vi "REACTOR_COMUNICACIONES.vi"(8 "error in (no error)":errorcluster) -> (0 "error out":errorcluster, 1 "COMMS":T1={"Alicats"="COM4", "Alic"=TRUE, "eValve"="COM6", "eval"=TRUE, "Eurotherm"="COM8", "euro"=TRUE, "Cell GAS"="COM10", "cgas"=TRUE, "Cell H2S"="COM5", "ch2s"=TRUE}, 2 "Cancelled?":bool)   [LabVIEW 2017]
doc: "Use this template to create a dialog box. This template polls the state of the buttons on the front panel and does not use events. Use the Dialog Using Events template (not available in Base package) to create a dialog box with event handling."
uses:
  REACTOR_COMUNICACIONES.ctl
panel:
  in  "Alic":bool=TRUE
  in  "Euro":bool=TRUE
  in  "V4v":bool=TRUE
  in  "Alicats":refnum<visa-resource-name>="COM4"
  in  "Eurotherm":refnum<visa-resource-name>="COM6"
  in  "EV4Posic":refnum<visa-resource-name>="COM7"
  out "Enable":bool=TRUE
  out "Disable":bool
  in  "Cancel":bool
  in  "OK":bool
  # "Comunicaciones"
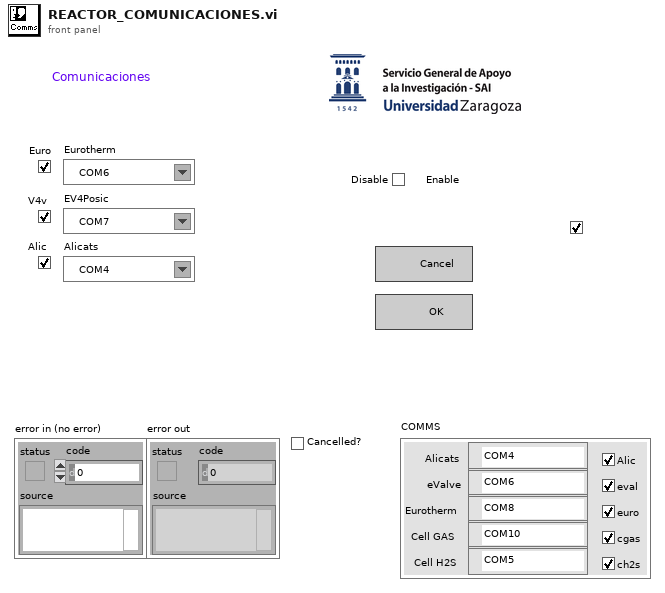
[diagram p1: front panel]
types:
  T1 = typedef "REACTOR_COMUNICACIONES.ctl" = cluster{"Alicats":refnum<visa-resource-name>, "Alic":bool, "eValve":refnum<visa-resource-name>, "eval":bool, "Eurotherm":refnum<visa-resource-name>, "euro":bool, "Cell GAS":refnum<visa-resource-name>, "cgas":bool, "Cell H2S":refnum<visa-resource-name>, "ch2s":bool}
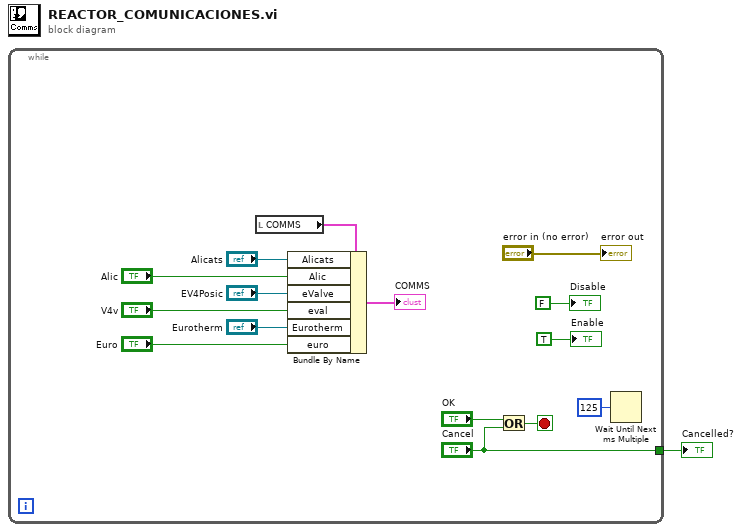
[diagram p0: block diagram]
diagram:
  n1 = while {
    tunnel: ["Cancel"] -> w1
    stop <- w15 stop-if-true
    n2 = local read "COMMS"() -> (w2:T1)
    n3 = Bundle By Name(cluster=w2, "Alicats"="Alicats", "Alic"="Alic", "eValve"="EV4Posic", "eval"="V4v", "Eurotherm"="Eurotherm", "euro"="Euro") -> (→"COMMS":T1)
    n4 = Or(x="OK", y="Cancel") -> (x .or. y?=w15:bool)
    n5 = Wait Until Next ms Multiple(millisecond multiple=u32 125) -> ()  [unwired: 1 out]
    "error out" <- "error in (no error)"
    "Disable" <- FALSE ("No usado")
    "Enable" <- TRUE ("Si usado")
  }
  "Cancelled?" <- w1
